vi "Using a Notifier As a Demultiplexer.vi"() -> ()   [LabVIEW 2023]
doc: "This VI shows the similarity between Notifiers and Demultiplexers. Demultiplex means \"one-to-many.\" Notifiers allow data to be sent to many locations from one data source. In this demo VI, a sine wave is sent to three data retrieval loops that all consume the data and run in parallel."
panel:
  out "Data Sink 3":dbl(graph)
  out "Data Sink 2":dbl(graph)
  in  "Stop":bool
  out "Data Sink 1":dbl(graph)
  # "Overview: Demonstrates the use of the Notifier functions to implement a demultiplexer.\nInstructions:\nRun the VI."
  # "These charts are in parallel loops, but they are all receiving their data from a single source notifier."
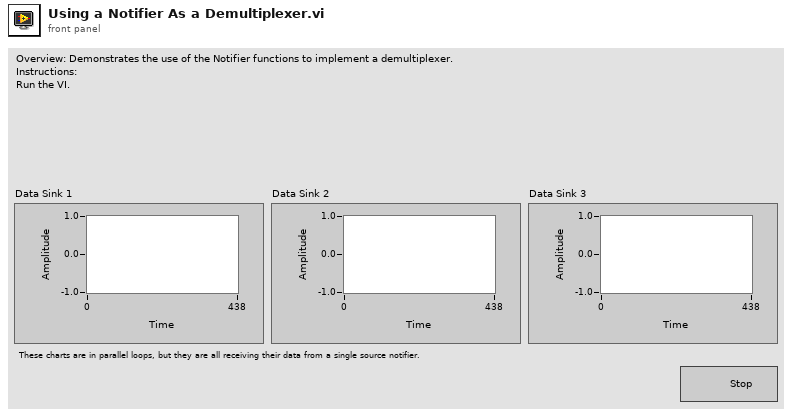
[diagram p1: front panel]
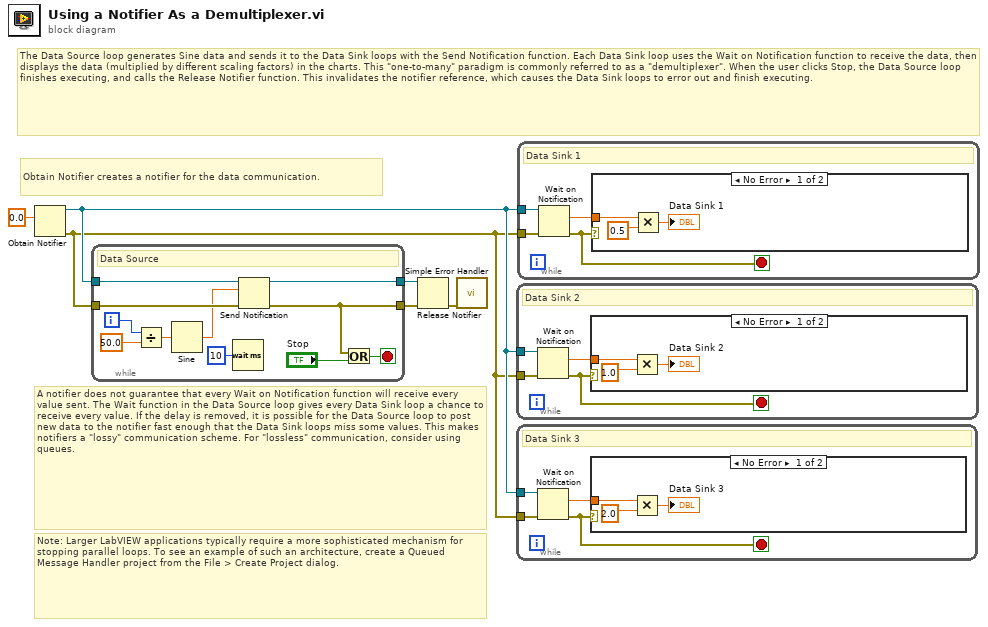
[diagram p0: block diagram]
diagram:
  # "Note: Larger LabVIEW applications typically require a more sophisticated mechanism for stopping parallel loops. To see an example of such an architecture, create a Queued Message Handler project from the File > Create Project dialog."
  # "Obtain Notifier creates a notifier for the data communication."
  # "The Data Source loop generates Sine data and sends it to the Data Sink loops with the Send Notification function. Each Data Sink loop uses the Wait on Notification function to receive the data, then displays the data (multiplied by different scaling factors) in the charts. This \"one-to-many\" paradigm is commonly referred to as a \"demultiplexer\". When the user clicks Stop, the Data Source loop finishes executing, and calls the Release Notifier function. This invalidates the notifier reference, which causes the Data Sink loops to error out and finish executing."
  # "A notifier does not guarantee that every Wait on Notification function will receive every value sent. The Wait function in the Data Source loop gives every Data Sink loop a chance to receive every value. If the delay is removed, it is possible for the Data Source loop to post new data to the notifier fast enough that the Data Sink loops miss some values. This makes notifiers a \"lossy\" communication scheme. For \"lossless\" communication, consider using queues."
  n1 = Obtain Notifier(notification data type=0.0) -> (notifier out=w3:refnum<notifier>, error out=w2:errorcluster)  [unwired: 3 in, 1 out]
  n2 = while "Data Source Loop" {
    tunnel: w3 -> [w17]
    tunnel: w2 -> [w16]
    tunnel: [w14] -> w6
    tunnel: [w7] -> w5
    i -> [w9]
    stop <- w13 stop-if-true
    # "Data Source"
    n3 = Divide(x=w9, y=50.0) -> (x/y=w10:dbl)
    n4 = Sine(x=w10) -> (sin(x)=w11:dbl)
    n5 = Wait (ms)(milliseconds to wait=u32 10 ("Time Between Iterations (ms)")) -> ()  [unwired: 1 out]
    n6 = Send Notification(notification=w11, notifier=w17, error in (no error)=w16) -> (notifier out=w14:refnum<notifier>, error out=w7:errorcluster)
    n7 = Or(x=w7, y="Stop") -> (x .or. y?=w13:bool)
  }
  n8 = Release Notifier(notifier=w6, error in (no error)=w5) -> (error out=w1:errorcluster)  [unwired: 1 in, 2 out]
  n9 = call <vilib>:"Simple Error Handler.vi"("error in (no error)"=w1) -> ()  [unwired: 4 in, 5 out]
  n10 = while "Data Sink One" {
    tunnel: w3 -> [w21]
    tunnel: w2 -> [w19]
    stop <- w18 stop-if-true
    # "Data Sink 2"
    n11 = Wait on Notification(notifier=w21, error in (no error)=w19) -> (notification=w20:dbl, error out=w18:errorcluster)  [unwired: 2 in, 2 out]
    n12 = case shown="No Error" w18 {
      tunnel: w20 -> [w24 _]
      frame No Error {
        n13 = Multiply(x=w24, y=1.0) -> (x*y=→"Data Sink 2":dbl)
      }
      frame Error {
      }
    }
  }
  n14 = while "Data Sink One" {
    tunnel: w3 -> [w28]
    tunnel: w2 -> [w26]
    stop <- w25 stop-if-true
    # "Data Sink 3"
    n15 = Wait on Notification(notifier=w28, error in (no error)=w26) -> (notification=w27:dbl, error out=w25:errorcluster)  [unwired: 2 in, 2 out]
    n16 = case shown="No Error" w25 {
      tunnel: w27 -> [w31 _]
      frame No Error {
        n17 = Multiply(x=w31, y=2.0) -> (x*y=→"Data Sink 3":dbl)
      }
      frame Error {
      }
    }
  }
  n18 = while "Data Sink One" {
    tunnel: w3 -> [w35]
    tunnel: w2 -> [w33]
    stop <- w32 stop-if-true
    # "Data Sink 1"
    n19 = Wait on Notification(notifier=w35, error in (no error)=w33) -> (notification=w34:dbl, error out=w32:errorcluster)  [unwired: 2 in, 2 out]
    n20 = case shown="No Error" w32 {
      tunnel: w34 -> [w38 _]
      frame No Error {
        n21 = Multiply(x=w38, y=0.5) -> (x*y=→"Data Sink 1":dbl)
      }
      frame Error {
      }
    }
  }
